vi "Wait_For_Notification.vi"(3 "Error In":errorcluster, 4 "Mode":enum16{"Position", "Velocity"}(ring), 5 "Serial In":refnum<visa-resource-name>) -> (0 "Error Out":errorcluster, 2 "Serial Out":refnum<visa-resource-name>)   [LabVIEW 2019]
uses:
  <vilib>/Instr/_visa.llb/Select Event Type.ctl
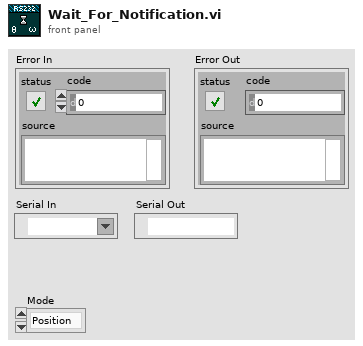
[diagram p1: front panel]
types:
  T1 = typedef "Select Event Type.ctl" = u32
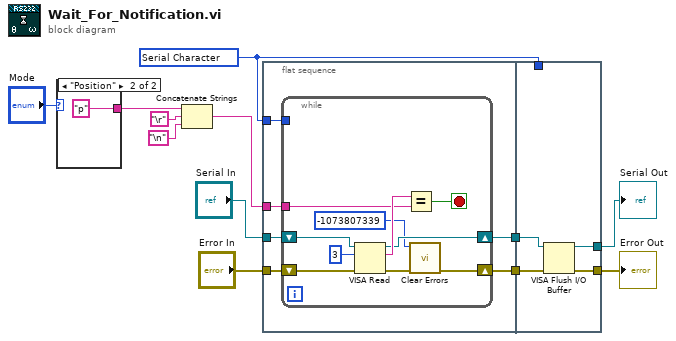
[diagram p0: block diagram]
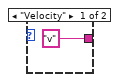
[diagram p2: hidden frame]
diagram:
  w7 = T1 1073684533 items=["Service Request"=1073684491, "Trigger"=3221168138, "Clear"=1073684493, "VXI Signal"=1073684512, "VXI/VME Interrupt"=3221168161, "VXI/VME Sysfail"=1073684509, "VXI/VME Sysreset"=1073684510, "GPIB CIC"=1073684498, "GPIB Talk"=1073684499, "GPIB Listen"=1073684500, "PXI Interrupt"=1073684514, "Serial Break"=1073684515, "Serial TermChar"=1073684516, "Serial CTS"=1073684521, "Serial DSR"=1073684522, "Serial DCD"=1073684524, "Serial RI"=1073684526, "Serial Character"=1073684533, "USB Interrupt"=1073684535, "All Enabled"=1073709055] ("Event Type")
  n1 = case shown="\"Position\"" "Mode" {
    tunnel: ["v" ("string") "p" ("string")] -> w11
    frame "Velocity" {
    }
    frame "Position" {
    }
  }
  n2 = Concatenate Strings(w11, "\r", "\n") -> (w10:string)
  n3 = flat-sequence {
    tunnel: w7 -> [w20]
    tunnel: w10 -> [w19]
    tunnel: [w18] -> w9
    tunnel: [w17] -> w8
    tunnel: "Error In" -> [w16]
    tunnel: "Serial In" -> [w15]
    tunnel: w9 -> [w32]
    tunnel: w8 -> [w31]
    tunnel: w7 -> [_]
    tunnel: [w34] -> w2
    tunnel: [w33] -> w1
    frame #0 {
      n4 = while {
        tunnel: w20 -> [_]
        tunnel: w19 -> [w28]
        shift-right: [w22] -> w17
        shift-left: w16 -> [w25]
        shift-right: [w26] -> w18
        shift-left: w15 -> [w24]
        stop <- w27 stop-if-true
        n5 = VISA Read(VISA resource name=w24, byte count=u32 3, error in (no error)=w25) -> (VISA resource name out=w26:refnum<visa-resource-name>, read buffer=w29:string, error out=w23:errorcluster)  [unwired: 1 out]
        n6 = Equal?(x=w29, y=w28) -> (x = y?=w27:bool)
        n7 = call <vilib>:"Clear Errors.vi"("error in (no error)"=w23, "specific error code to clear (0: all)"=-1073807339) -> ("error out"=w22:errorcluster)  [unwired: 4 in, 1 out]
      }
    }
    frame #1 {
      n8 = VISA Flush I/O Buffer(VISA resource name=w32, error in (no error)=w31) -> (VISA resource name out=w34:refnum<visa-resource-name>, error out=w33:errorcluster)  [unwired: 1 in]
    }
  }
  "Error Out" <- w1
  "Serial Out" <- w2
